vi "library_path.vi"() -> (3 "path out":path)   [LabVIEW 2019, in "MSCU.lvclass"]
uses:
  MSCU.lvclass
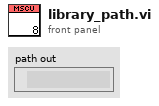
[diagram p1: front panel]
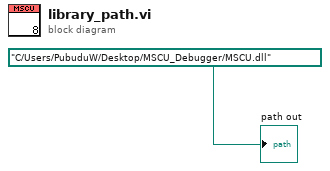
[diagram p0: block diagram]
diagram:
  "path out" <- path "C:/Users/PubuduW/Desktop/MSCU_Debugger/MSCU.dll" ("path in")
